vi "AVS_OneReading.vi"(4 "error in (no error) 4":errorcluster, 7 "AVS-VISA":refnum<visa-resource-name>) -> (0 "error out (no error)":errorcluster, 2 "AVS Resistance reading":dbl format="%.2f", 3 "dup AVS-VISA":refnum<visa-resource-name>)   [LabVIEW 2019]
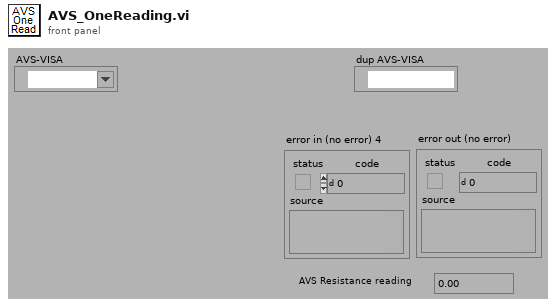
[diagram p1: front panel]
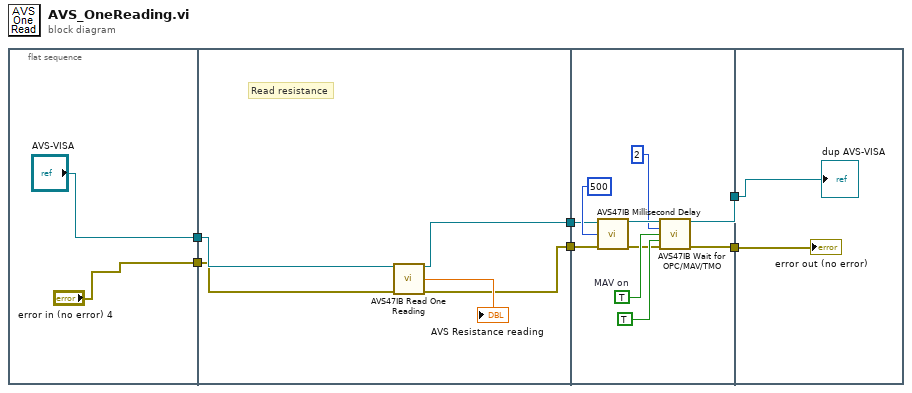
[diagram p0: block diagram]
diagram:
  n1 = flat-sequence {
    tunnel: ["AVS-VISA"] -> w6
    tunnel: ["error in (no error) 4"] -> w5
    tunnel: w6 -> [w13]
    tunnel: w5 -> [w12]
    tunnel: [w10] -> w4
    tunnel: [w9] -> w2
    tunnel: w4 -> [w18]
    tunnel: [w17] -> w3
    tunnel: w2 -> [w16]
    tunnel: [w15] -> w1
    tunnel: w3 -> [w24]
    tunnel: w1 -> [w25]
    frame #0 {
    }
    frame #1 {
      # "Read resistance"
      n2 = call "AVS47IB Read One Reading.vi"("VISA session"=w13, "error in (no error)"=w12) -> ("dup VISA session"=w10:refnum<visa-resource-name>, "Resistance reading"=→"AVS Resistance reading":dbl, "error out"=w9:errorcluster)  [unwired: 9 in, 2 out]
    }
    frame #2 {
      w23 = TRUE  # MAV on
      n3 = call "AVS47IB Millisecond Delay.vi"("VISA session"=w18, "Delay (50 ms)"=u32 500, "error in (no error)"=w16) -> ("dup VISA session"=w21:refnum<visa-resource-name>, "error out"=w20:errorcluster)  [unwired: 11 in]
      n4 = call "AVS47IB Wait for OPC/MAV/TMO.vi"("VISA session"=w21, "Timeout (2 sec)"=i16 2, "MAV (on)"=w23, "OPC (off)"=TRUE, "error in (no error)"=w20) -> ("dup VISA session"=w17:refnum<visa-resource-name>, "error out"=w15:errorcluster)  [unwired: 8 in, 1 out]
    }
    frame #3 {
      "error out (no error)" <- w25
      "dup AVS-VISA" <- w24
    }
  }
